vi "Ave MIN Query.vi"(8 "error in (no error)":errorcluster, 11 "VISA resource name":refnum<visa-resource-name>) -> (0 "error out":errorcluster, 2 "Measurement":dbl, 3 "VISA resource name out":refnum<visa-resource-name>)   [LabVIEW 2017, in "ADCMT7451_ADC.lvlib"]
doc: "Queries the result of Max/Min calculation."
uses:
  ADCMT7451_ADC.lvlib
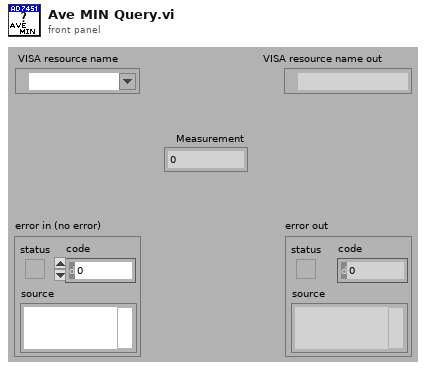
[diagram p1: front panel]
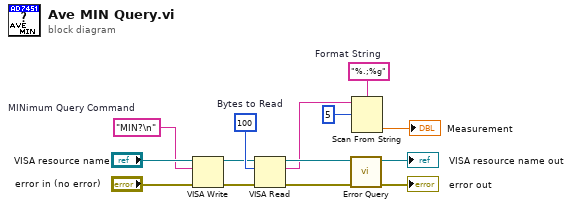
[diagram p0: block diagram]
diagram:
  w4 = "%.;%g"  # Format String
  w10 = "MIN?\n"  # MINimum Query Command
  w13 = u32 100  # Bytes to Read
  n1 = VISA Write(VISA resource name="VISA resource name", write buffer=w10, error in (no error)="error in (no error)") -> (VISA resource name out=w12:refnum<visa-resource-name>, error out=w11:errorcluster)  [unwired: 1 out]
  n2 = VISA Read(VISA resource name=w12, byte count=w13, error in (no error)=w11) -> (VISA resource name out=w8:refnum<visa-resource-name>, read buffer=w2:string, error out=w9:errorcluster)  [unwired: 1 out]
  n3 = call "Error Query.vi"("error in (no error)"=w9, "VISA resource name"=w8) -> ("error out"=→"error out":errorcluster, "VISA resource name out"=→"VISA resource name out":refnum<visa-resource-name>)  [unwired: 6 in, 2 out]
  n4 = Scan From String(format string=w4, input string=w2, initial scan location=5) -> (output 1=→"Measurement":dbl)  [unwired: 2 in, 3 out]
